vi "MenuBuild.vi"(4 "Button\n(Mouse Down?)":u16, 5 "Clipboard":refnum<vi>, 6 "withinSelection?":bool=TRUE, 7 "row type":T1, 8 "error in (no error)":errorcluster, 9 "Table CtlRef In":refnum<vi>, 10 "MenuRef In":refnum<k9>, 11 "DigitalCol in":refnum<class "DigitalCol.lvclass">) -> (0 "error out":errorcluster, 1 "Table CtlRef Out":refnum<vi>, 2 "MenuRef Out":refnum<k9>, 3 "DigitalCol out":refnum<class "DigitalCol.lvclass">)   [LabVIEW 2013, in "DigitalCol.lvclass"]
doc: "Build shortcut (right-click) menu items for digital columns. This VI is read-only w.r.t column data."
uses:
  DigitalCol.lvclass
  TypeDefs/RowType.ctl
  Column/Column.lvclass
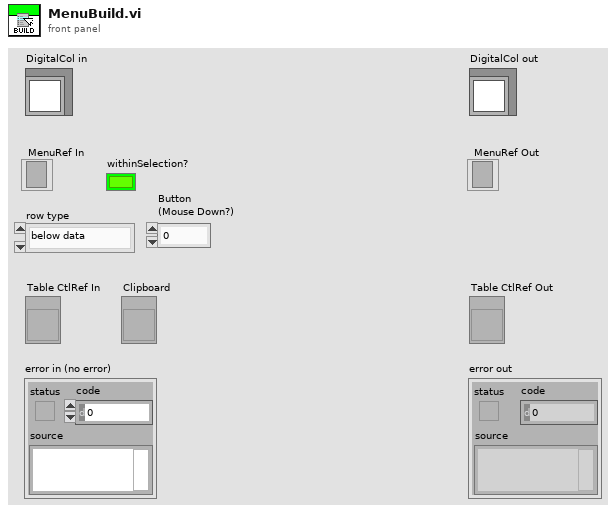
[diagram p1: front panel]
types:
  T1 = typedef "RowType.ctl" = enum16{"below data", "within data", "column header", "first row"}
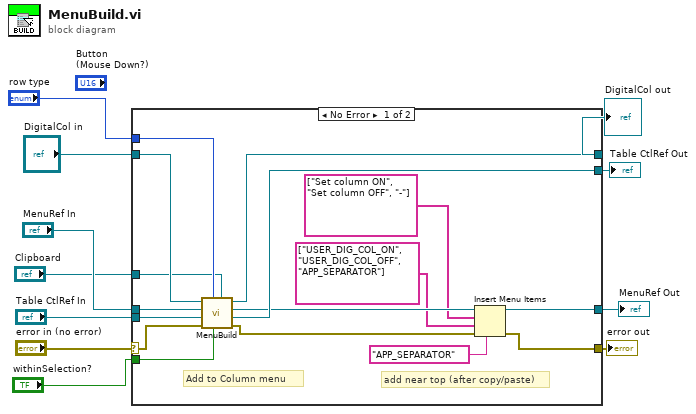
[diagram p0: block diagram]
diagram:
  n1 = case shown="No Error" "error in (no error)" {
    selector: "error in (no error)" -> [w21 w31]
    tunnel: [w27 w28] -> w11
    tunnel: [w20 w29] -> w10
    tunnel: [w26 w30] -> w9
    tunnel: "row type" -> [w25 _]
    tunnel: "Table CtlRef In" -> [w24 w28]
    tunnel: "MenuRef In" -> [w23 w29]
    tunnel: "DigitalCol in" -> [w22 w30]
    tunnel: [w17 w31] -> w4
    tunnel: "withinSelection?" -> [w14 _]
    tunnel: "Clipboard" -> [w12 _]
    frame No Error {
      # "Add to Column menu"
      # "add near top (after copy/paste)"
      n2 = call-parent "MenuBuild.vi"("Clipboard"=w12, "withinSelection?"=w14, "row type"=w25, "error in (no error)"=w21, "Table CtlRef In"=w24, "MenuRef In"=w23, "Column in"=w22) -> ("error out"=w18:errorcluster, "Table CtlRef Out"=w27:refnum<vi>, "MenuRef Out"=w19:refnum<k9>, "Column out"=w26:refnum<class "DigitalCol.lvclass">)  [unwired: 1 in]
      n3 = Insert Menu Items(4:"APP_SEPARATOR" ("after item"), 6:w18, 7:string[] ["USER_DIG_COL_ON", "USER_DIG_COL_OFF", "APP_SEPARATOR"], 8:string[] ["Set column ON", "Set column OFF", "-"], 9:w19) -> (0:w17:errorcluster, 3:w20:refnum<k9>)  [unwired: 1 in, 1 out]
    }
    frame Error {
    }
  }
  "error out" <- w4
  "DigitalCol out" <- w9
  "MenuRef Out" <- w10
  "Table CtlRef Out" <- w11
